vi "B7_72_CheckMode.vi"(4 "Error Code":T8=5490, 5 "Delay Time (s)":T6=0.5, 6 "Driver Name":T9="B1_28", 7 "Mode2check":T7="U4", 8 "error in":T10, 11 "DriverConnect in":T1={"InterfaceType"=enum."VISA", "OpenedSession"="", "InterfaceSettings"={"Interface"=enum."RS232", "EOS 4 read"=enum."LF (\\n)", "EOS 4 write"=enum."LF (\\n)", "TMO, ms"=10000, "Sett"=variant(cluster{"Baud Rate":u32, "Data Bits":u16, "Parity":u16, "Stop Bits":u16, "Flow Control":u16, "Eho":bool} {"Baud Rate"=75, "Data Bits"=0, "Parity"=0, "Stop Bits"=0, "Flow Control"=0, "Eho"=FALSE})}}) -> (0 "error out":T10, 3 "DriverConnect out":T1={"InterfaceType"=enum."VISA", "OpenedSession"="", "InterfaceSettings"={"Interface"=enum."RS232", "EOS 4 read"=enum."LF (\\n)", "EOS 4 write"=enum."LF (\\n)", "TMO, ms"=10000, "Sett"=variant(cluster{"Baud Rate":u32, "Data Bits":u16, "Parity":u16, "Stop Bits":u16, "Flow Control":u16, "Eho":bool} {"Baud Rate"=75, "Data Bits"=0, "Parity"=0, "Stop Bits"=0, "Flow Control"=0, "Eho"=FALSE})}})   [LabVIEW 2018]
uses:
  MOKO_LabViewLibrary/MokoLowLevel/MokoLowLovelControl/MLLC_Error.ctl
  MOKO_LabViewLibrary/MokoLowLevel/MokoLowLovelControl/MLLC_DriverName.ctl
  MOKO_LabViewLibrary/MokoLowLevel/MokoLowLovelControl/MLLC_ErrorCode.ctl
  MOKO_LabViewLibrary/MokoLowLevel/MokoLowLovelControl/MLLC_Command.ctl
  MOKO_LabViewLibrary/MokoLowLevel/MokoLowLovelControl/MLLC_Delay.ctl
  MOKO_LabViewLibrary/MokoLowLevel/MokoLowLovelControl/MLLC_ConnectCluster.ctl
  MOKO_LabViewLibrary/MokoLowLevel/MokoLowLovelControl/MLLC_InterfaceType.ctl
  MOKO_LabViewLibrary/MokoLowLevel/MokoLowLovelControl/MLLC_OpenedSession.ctl
  MOKO_LabViewLibrary/MokoLowLevel/MokoLowLovelControl/MLLC_InterfaceSettings.ctl
  MOKO_LabViewLibrary/MokoLowLevel/MokoLowLovelControl/MLLC_InterfaceKind.ctl
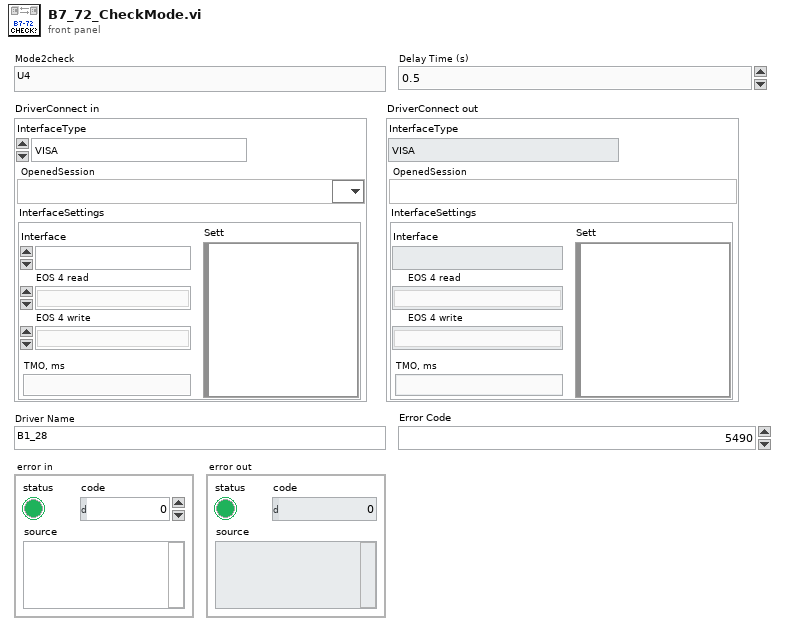
[diagram p1: front panel]
types:
  T1 = typedef "MLLC_ConnectCluster.ctl" = cluster{"InterfaceType":T2, "OpenedSession":T3, "InterfaceSettings":T4}
  T2 = typedef "MLLC_InterfaceType.ctl" = enum16{"VISA", "Prologix USB-GPIB"}
  T3 = typedef "MLLC_OpenedSession.ctl" = refnum<visa-resource-name>
  T4 = typedef "MLLC_InterfaceSettings.ctl" = cluster{"Interface":T5, "EOS 4 read":enum16{"Default (=EOS 4 write)", "CR (\\r)", "LF (\\n)", "None"}, "EOS 4 write":enum16{"CR+LF (\\r\\n)", "CR (\\r)", "LF (\\n)", "None"}, "TMO, ms":i32, "Sett":variant}
  T5 = typedef "MLLC_InterfaceKind.ctl" = enum16{"RS232", "GPIB", "USB", "Ethernet", "another"}
  T6 = typedef "MLLC_Delay.ctl" = dbl
  T7 = typedef "MLLC_Command.ctl" = string
  T8 = typedef "MLLC_ErrorCode.ctl" = u32
  T9 = typedef "MLLC_DriverName.ctl" = string
  T10 = typedef "MLLC_Error.ctl" = errorcluster
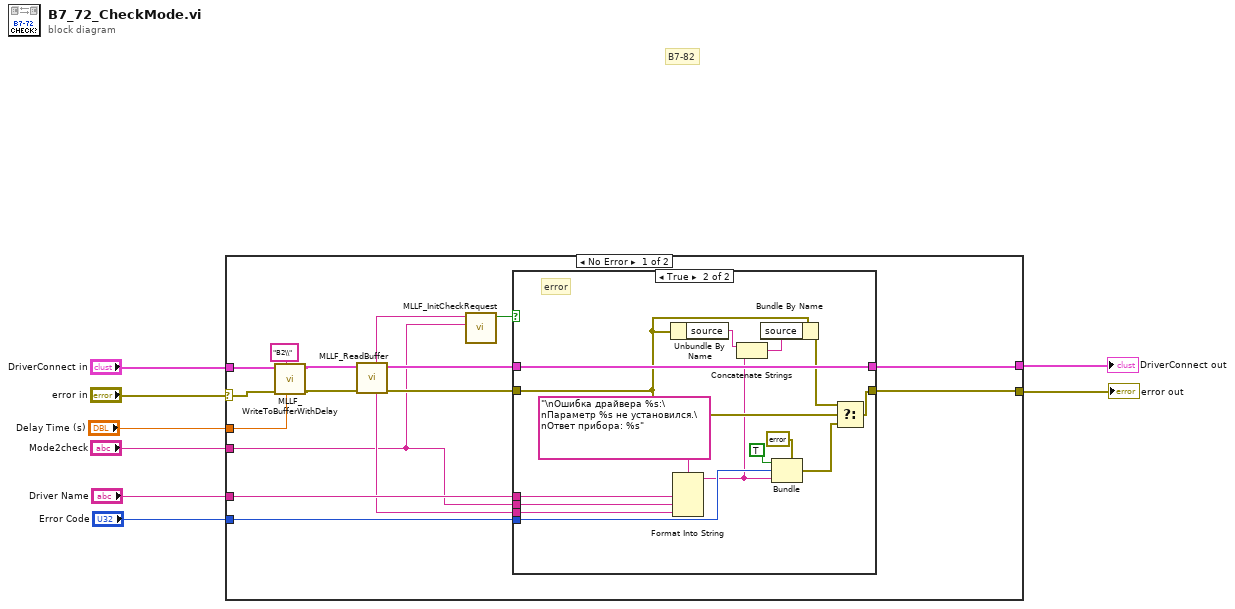
[diagram p0: block diagram]
diagram:
  # "B7-82"
  n1 = case shown="No Error" "error in" {
    selector: "error in" -> [w23 w42]
    tunnel: [w13 w42] -> w8
    tunnel: "Driver Name" -> [w18 _]
    tunnel: "Error Code" -> [w17 _]
    tunnel: [w14 w41] -> w1
    tunnel: "Mode2check" -> [w9 _]
    tunnel: "Delay Time (s)" -> [w22 _]
    tunnel: "DriverConnect in" -> [w12 w41]
    frame No Error {
      n2 = call "MLLF_WriteToBufferWithDelay.vi"("Delay Time ( 0,05 s)"=w22, "Command"="B2\\" ("String"), "Error In"=w23, "DriverConnect in"=w12) -> ("Error Out"=w20:errorcluster, "DriverConnect out"=w21:T1)  [unwired: 6 in]
      n3 = call "MLLF_ReadBuffer.vi"("Error In"=w20, "DriverConnect in"=w21) -> ("Error Out"=w15:errorcluster, "DriverConnect out"=w16:T1, "String"=w10:string)  [unwired: 6 in]
      n4 = call "MLLF_InitCheckRequest.vi"("Answer"=w9, "Response Init"=w10) -> ("Design"=w11:bool)  [unwired: 6 in, 3 out]
      n5 = case shown="True" w11 {
        tunnel: w16 -> [w25 w34]
        tunnel: [w25 w34] -> w14
        tunnel: [w24 w26] -> w13
        tunnel: w15 -> [w24 w32]
        tunnel: w9 -> [_ w35]
        tunnel: w17 -> [_ w37]
        tunnel: w18 -> [_ w36]
        tunnel: w10 -> [_ w33]
        frame False {
          # "no error"
        }
        frame True {
          # "error"
          n6 = Unbundle By Name(w32) -> ("source"=w31:string)
          n7 = Format Into String(format string="\nОшибка драйвера %s:\nПараметр %s не установился.\nОтвет прибора: %s", w36, w35, w33) -> (resulting string=w29:string)  [unwired: 2 in, 1 out]
          n8 = Concatenate Strings(w31, w29) -> (w30:string)
          n9 = Bundle By Name(cluster=w32, "source"=w30) -> (w28:errorcluster)
          n10 = Bundle(cluster=errorcluster {"status"=FALSE, "code"=0, "source"=""} ("error out"), "status"=TRUE ("Status"), "code"=w37, "source"=w29) -> (w27:errorcluster)
          n11 = Select(t=w28, s=w32, f=w27) -> (s? t:f=w26:errorcluster)
        }
      }
    }
    frame Error {
    }
  }
  "error out" <- w8
  "DriverConnect out" <- w1
